vi "AV Write Array.vi"(8 "error in":errorcluster, 10 "Temperature AV":dbl[](array[numeric]), 11 "Temperature Actual Value in":refnum<class "Temperature Actual Value.lvclass">) -> (0 "error out":errorcluster, 3 "Temperature Actual Value out":refnum<class "Temperature Actual Value.lvclass">)   [LabVIEW 2023, in "Temperature Actual Value.lvclass"]
uses:
  Temperature Actual Value.lvclass
  Parents/Actual Value/Actual Value.lvclass
  Temperature Actual Value.lvclass/Temperature Actual Value.ctl
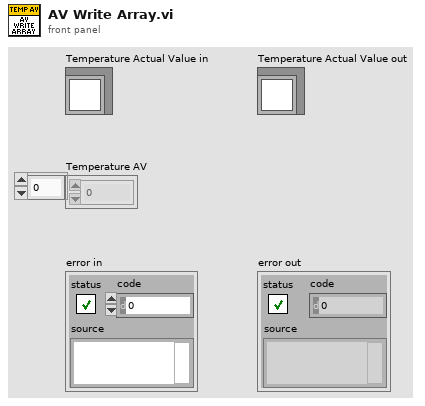
[diagram p1: front panel]
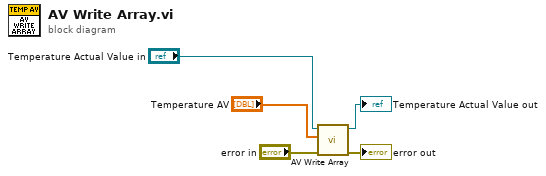
[diagram p0: block diagram]
diagram:
  n1 = call-parent "AV Write Array.vi"("error in"="error in", "Actual Value"="Temperature AV", "Actual Value in"="Temperature Actual Value in") -> ("error out"=→"error out":errorcluster, "Actual Value out"=→"Temperature Actual Value out":refnum<class "Temperature Actual Value.lvclass">)  [unwired: 7 in]
